vi "Stop Core.vi"(10 "final error code":i32, 11 "TCP_Client_Window in":refnum<class "TCP_Client_Window.lvclass">) -> (3 "TCP_Client_Window out":refnum<class "TCP_Client_Window.lvclass">)   [LabVIEW 2023, in "TCP_Client_Window.lvlib" / "TCP_Client_Window.lvclass"]
doc: "(<B>Filename</B>: Actor Framework.lvlib:Actor.lvclass:Stop Core.vi)\n\nDefines what the actor does before it stops. Use the <B>final error code</B> input to determine whether the actor shut down in response to an error.\n\nBy default, this method passes the Stop message along to all auto-stop nested actors. A descendant class may override this method to define additional behavior, such as shutting down any processes the actor initiated in its override of the Actor Core method."
uses:
  TCP_Client_Window.lvclass
  TCP_Client_Window.lvclass/TCP_Client_Window.ctl
  <vilib>/ActorFramework/Actor/Actor.lvclass
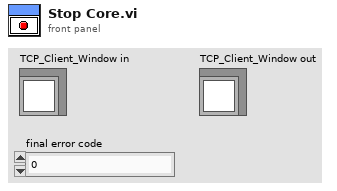
[diagram p1: front panel]
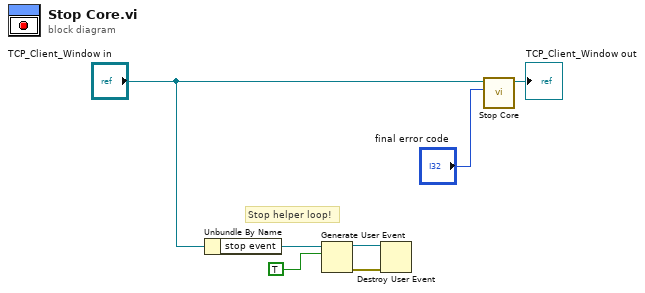
[diagram p0: block diagram]
diagram:
  # "Stop helper loop!"
  n1 = Unbundle By Name("TCP_Client_Window in") -> ("stop event"=w4:refnum<user-event>)
  n2 = Generate User Event(user event=w4, event data cluster=TRUE ("event data")) -> (user event out=w2:refnum<user-event>, error out=w3:errorcluster)  [unwired: 2 in]
  n3 = Destroy User Event(user event=w2, error in=w3) -> ()  [unwired: 1 out]
  n4 = call-parent "Stop Core.vi"("final error code"="final error code", "Actor in"="TCP_Client_Window in") -> ("Actor out"=→"TCP_Client_Window out":refnum<class "TCP_Client_Window.lvclass">)  [unwired: 9 in]
